vi "Play2 sounds.vi"(0 "error out":errorcluster, 8 "error in (no error)":errorcluster, 10 "path 2":path, 11 "path":path) -> ()   [LabVIEW 2010]
uses:
  <vilib>/sound2/lvsound2.llb/Sound File Read Open.vi
  <vilib>/sound2/lvsound2.llb/Sound File Info (path).vi
  <vilib>/sound2/lvsound2.llb/Sampling Mode.ctl
  <vilib>/sound2/lvsound2.llb/Sound File Position.ctl
  <vilib>/sound2/lvsound2.llb/Sound File Read (DBL).vi
  <vilib>/sound2/lvsound2.llb/Sound Output Write (DBL).vi
panel:
  in  "Start Position (Samples)":i32
  in  "Samples Per Read":i32=2000
  out "Read Position (Samples)":i32=364000
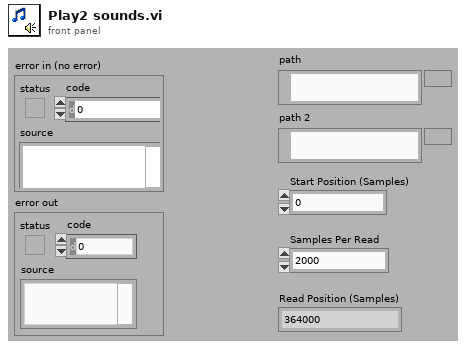
[diagram p1: front panel]
types:
  T1 = typedef "Sampling Mode.ctl" = i32
  T2 = typedef "Sound Data Format.ctl" = cluster{"sample rate (S/s)":dbl, "number of channels":i32, "bits per sample":i32}
  T3 = typedef "Sound File Refnum.ctl" = refnum<file>
  T4 = typedef "Sound Output Task ID.ctl" = u32
  T5 = typedef "Sound File Position.ctl" = u16
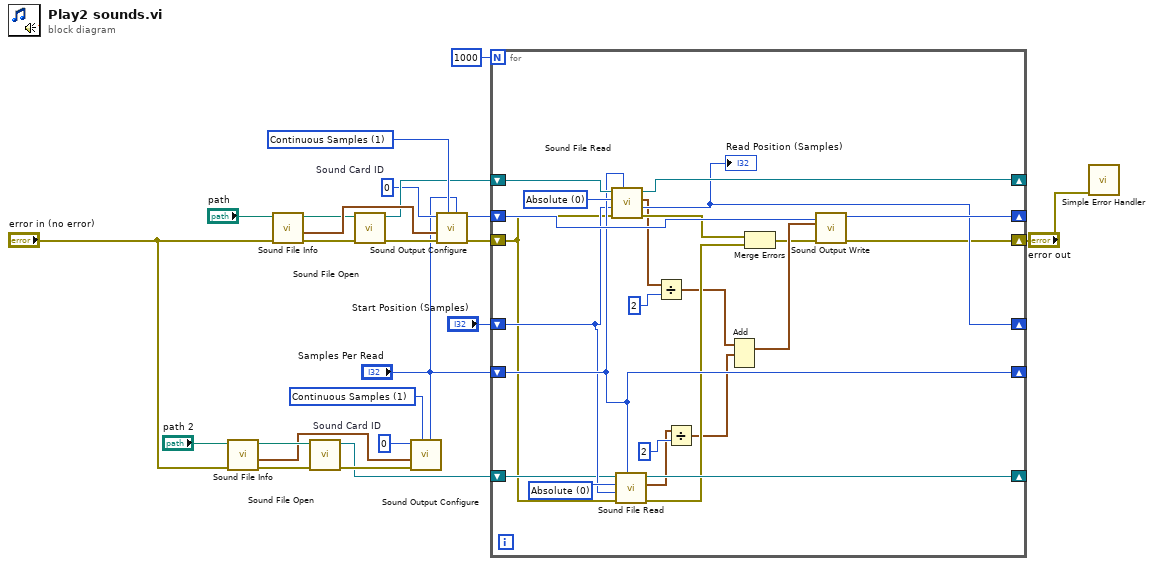
[diagram p0: block diagram]
diagram:
  w6 = T1 1 items=["Finite Samples", "Continuous Samples"] ("sample mode")
  w10 = u32 0  # Sound Card ID
  w22 = T1 1 items=["Finite Samples", "Continuous Samples"] ("sample mode")
  w13 = u32 0  # Sound Card ID
  n1 = call-poly <vilib>:"Sound File Info.vi"("error in (no error)"="error in (no error)", "path"="path 2") -> ("error out"=w7:errorcluster, "sound format"=w5:T2, "path out"=w9:path)  [unwired: 6 in, 1 out]
  n2 = call-poly <vilib>:"Sound File Info.vi"("error in (no error)"="error in (no error)", "path"="path") -> ("error out"=w19:errorcluster, "sound format"=w23:T2, "path out"=w17:path)  [unwired: 6 in, 1 out]
  n3 = call-poly <vilib>:"Sound File Open.vi"("error in (no error)"=w7, "path"=w9) -> ("error out"=w8:errorcluster, "sound file refnum"=w1:T3)  [unwired: 8 in]
  n4 = call-poly <vilib>:"Sound File Open.vi"("error in (no error)"=w19, "path"=w17) -> ("error out"=w18:errorcluster, "sound file refnum"=w20:T3)  [unwired: 8 in]
  n5 = call <vilib>:"Sound Output Configure.vi"("number of samples/ch"="Samples Per Read", "sample mode"=w6, "error in (no error)"=w8, "sound format"=w5, "device ID"=w10) -> ()  [unwired: 5 in, 2 out]
  n6 = call <vilib>:"Sound Output Configure.vi"("number of samples/ch"="Samples Per Read", "sample mode"=w22, "error in (no error)"=w18, "sound format"=w23, "device ID"=w13) -> ("error out"=w15:errorcluster, "task ID"=w21:T4)  [unwired: 5 in]
  n7 = for {
    N: 1000 -> [_]
    shift-right: [w42] -> _
    shift-left: w21 -> [w43]
    shift-right: [w40] -> w14
    shift-left: w15 -> [w33]
    shift-right: [w44] -> _
    shift-left: w20 -> [w46]
    shift-right: [w37] -> _
    shift-left: "Samples Per Read" -> [w37]
    shift-right: [w41] -> _
    shift-left: "Start Position (Samples)" -> [w36]
    shift-right: [w34] -> _
    shift-left: w1 -> [w35]
    w38 = T5 0 items=["Absolute"=0, "Relative"=2] ("position mode")
    w45 = T5 0 items=["Absolute"=0, "Relative"=2] ("position mode")
    n8 = call-poly <vilib>:"Sound File Read.vi"("number of samples/ch (-1: all)"=w37, "error in (no error)"=w33, "position offset"=w36, "position mode"=w45, "sound file refnum"=w46) -> ("error out"=w31:errorcluster, "offset"=w41:i32, "data"=w29:waveform(dbl)[], "sound file refnum out"=w44:T3)  [unwired: 2 in, 1 out]
    "Read Position (Samples)" <- w41
    n9 = call-poly <vilib>:"Sound File Read.vi"("number of samples/ch (-1: all)"=w37, "error in (no error)"=w33, "position offset"=w36, "position mode"=w38, "sound file refnum"=w35) -> ("error out"=w30:errorcluster, "data"=w25:waveform(dbl)[], "sound file refnum out"=w34:T3)  [unwired: 2 in, 2 out]
    n10 = Divide(x=w29, y=2) -> (x/y=w27:waveform(dbl)[])
    n11 = Divide(x=w25, y=2) -> (x/y=w24:waveform(dbl)[])
    n12 = Add(1:w24, 2:w27) -> (0:w39:waveform(dbl)[])  [unwired: 1 in, 1 out]
    n13 = Merge Errors(w31, w30) -> (w32:errorcluster)
    n14 = call-poly <vilib>:"Sound Output Write.vi"("error in (no error)"=w32, "data"=w39, "task ID"=w43) -> ("error out"=w40:errorcluster, "task ID out"=w42:T4)  [unwired: 7 in]
  }
  n15 = call <vilib>:"Simple Error Handler.vi"("error in (no error)"=w14) -> ()  [unwired: 4 in, 5 out]
